vi "Read U32.vi"(8 "error in (no error)":errorcluster, 11 "Event in":refnum<class "Event U32.lvclass">) -> (0 "error out":errorcluster, 2 "U32":u32, 3 "Event out":refnum<class "Event U32.lvclass">)   [LabVIEW 2017, in "Event Actors.lvlib" / "Event U32.lvclass"]
uses:
  Event U32.lvclass
  Event U32.lvclass/Event U32.ctl
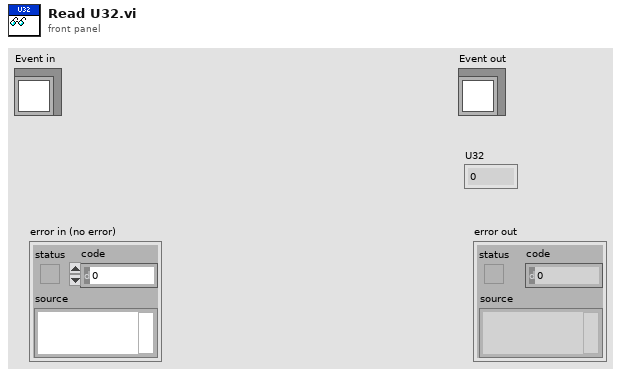
[diagram p1: front panel]
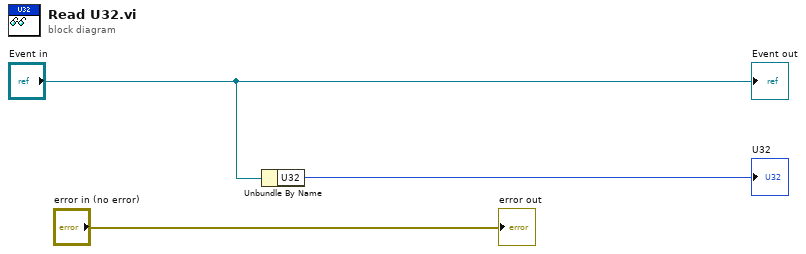
[diagram p0: block diagram]
diagram:
  n1 = Unbundle By Name("Event in") -> ("U32"=→"U32":u32)
  "Event out" <- "Event in"
  "error out" <- "error in (no error)"
